vi "Get Assertion Type From Test Case.vi"(8 "error in (no error)":errorcluster, 11 "Test Case Test Double in":refnum<class "Test Case Test Double.lvclass">) -> (0 "error out":errorcluster, 3 "Assertion Type":T1)   [LabVIEW 2020, in "LUnit Tests.lvlib" / "Assertion Result Test.lvclass"]
uses:
  Assertion Result Test.lvclass
  source/Framework/Result Classes/Assertion Result/Public/TypeDefs/Assertion Type.ctl
  Test Dummys/Test Case Test Double/Test Case Test Double.lvclass
  C:/Users/anton/Documents/GitHub/LUnit/source/Framework/Test Case/LUnit Test Case.lvclass
  source/Framework/Test Case/LUnit Test Case.lvclass/LUnit Test Case.ctl
  source/Framework/Result Classes/Test Case Result/Test Case Result.lvclass/Test Case Result.ctl
  source/Framework/Result Classes/Method Result/Method Result.lvclass/Method Result.ctl
  source/Framework/Result Classes/Assertion Result/Assertion Result.lvclass/Assertion Result.ctl
  source/Framework/Test Case/LUnit Test Case.lvclass
  source/Framework/Result Classes/Test Case Result/Test Case Result.lvclass
  source/Framework/Result Classes/Assertion Result/Assertion Result.lvclass
  source/Framework/Result Classes/Method Result/Method Result.lvclass
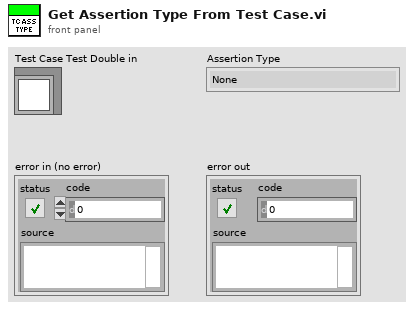
[diagram p1: front panel]
types:
  T1 = typedef "Assertion Result.lvclass/Assertion Type.ctl" = enum16{"None", "Pass", "Fail", "Skip", "Pass if Equal", "Fail if Equal", "Pass if Error", "Fail if Error", "Pass if", "Fail if"}
  T2 = map{string, refnum<class "Method Result.lvclass">}
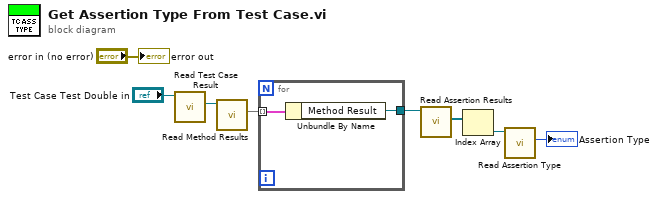
[diagram p0: block diagram]
diagram:
  n1 = call "Read Test Case Result.vi"("LUnit Test Case In"="Test Case Test Double in") -> ("Test Case Result"=w3:refnum<class "Test Case Result.lvclass">)  [unwired: 9 in, 1 out]
  n2 = call "Read Method Results.vi"("Test Case Result In"=w3) -> ("Method Results"=w4:T2)  [unwired: 9 in, 1 out]
  n3 = for {
    tunnel: [w9] -> w5
    tunnel: w4 -> [w10] mode=indexing
    n4 = Unbundle By Name(w10) -> ("Method Result"=w9:refnum<class "Method Result.lvclass">)
  }
  n5 = call "Read Assertion Results.vi"("Method Result In"=w5) -> ("Assertion Results"=w6:refnum<class "Assertion Result.lvclass">[])  [unwired: 9 in, 1 out]
  n6 = Index Array(array=w6) -> (element=w7:refnum<class "Assertion Result.lvclass">)  [unwired: 1 in]
  n7 = call "Read Assertion Type.vi"("Test Assertion Result In"=w7) -> ("Assertion Type"=→"Assertion Type":T1)  [unwired: 9 in, 1 out]
  "error out" <- "error in (no error)"
